vi "Agilent 428X Series Measure Capacitor D Value.vi"(7 "Voltage Level (V)(1.0V)":dbl=1.0 min=0.0 max=20.0 step=0.1 format="%.4f", 8 "error in (no error)":errorcluster, 9 "Freq Value (Hz)(1.0 MHz)":dbl=1000000.0 min=20.0 max=30000000.0 step=10.0 format="%.4e", 10 "Imp Type (0: CPD)":u32(ring) items=["CPD", "CPQ", "CPG", "CPRP", "CSD", "CSQ", "CSRS", "LPQ", "LPD", "LPG", "LPRP", "LSD", "LSQ", "LSRS", "RX", "ZTD", "ZTR", "GB", "YTD", "YTR"], 11 "VISA resource name":refnum<visa-resource-name>) -> (0 "error out":errorcluster, 1 "Secondary Value":dbl format="%^.4e", 2 "Primary Value":dbl format="%^.4e", 3 "VISA resource name out":refnum<visa-resource-name>, 4 "Data Status":bool=TRUE)   [LabVIEW 2015]
doc: "This VI is an example of how to use the HP428XA subVIs programmatically. This VI first configures a measurement, sets triggering, then takes measurements.\n\nThis function demonstrate one type of impedance measurement that can be made with the HP428XA and it accessories. In this example a 220 pF ceramic capacitor will be measured under the following conditions.\n\n DUT:\n 220 pF ceramic capacitor\n (HP Part Number 0160-4812)\n\n Measurement Conditions: \n \n Function: Cp-D\n Frequency: 1.0 MHz\n Test Signal Level: 1.0 V\n \n Equipment Required:\n\n HP 16047C Test Fixture\n Shorting bar (HP Part Number 5000-4226) or equivalent\n\nNote:\nFor more details see to the operation manual in Chapter 3."
uses:
  <instrlib>/Agilent 428X Series/Agilent 428X Series.lvlib
panel:
  # "© Copyright 2005 National Instruments Corporation.  All Rights Reserved."
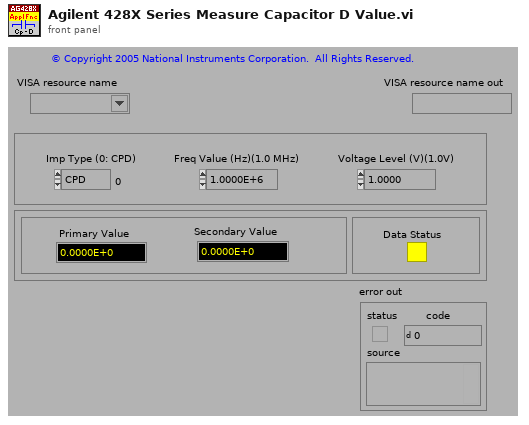
[diagram p1: front panel]
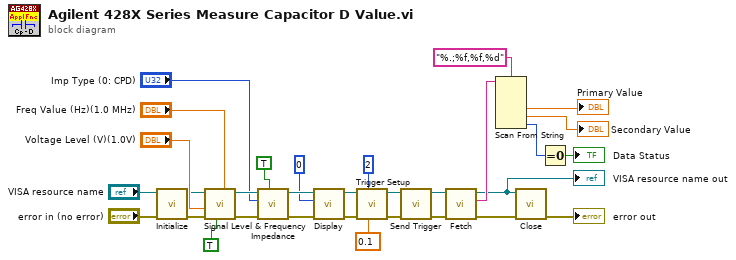
[diagram p0: block diagram]
diagram:
  n1 = call <instrlib>:"Initialize.vi"("error in (no error)"="error in (no error)", "VISA resource name"="VISA resource name") -> ("error out"=w5:errorcluster, "VISA resource name out"=w4:refnum<visa-resource-name>)  [unwired: 8 in]
  n2 = call <instrlib>:"Signal Level & Frequency.vi"("Frequency Value (Hz) (100KHz)"="Freq Value (Hz)(1.0 MHz)", "Oscillator Select (T: Voltage)"=TRUE, "error in (no error)"=w5, "Voltage Level (V) (5mV)"="Voltage Level (V)(1.0V)", "VISA resource name"=w4) -> ("error out"=w23:errorcluster, "VISA resource name out"=w31:refnum<visa-resource-name>)  [unwired: 5 in]
  n3 = call <instrlib>:"Impedance.vi"("Auto Range (F: Off)"=TRUE ("Auto Range (Off:F)"), "error in (no error)"=w23, "Imp Type (0: CPD)"="Imp Type (0: CPD)", "VISA resource name"=w31) -> ("error out"=w24:errorcluster, "VISA resource name out"=w30:refnum<visa-resource-name>)  [unwired: 6 in]
  n4 = call <instrlib>:"Display.vi"("error in (no error)"=w24, "Display Page (0: Measurement)"=u32 0 ("Display Page (Measurment:0)"), "VISA resource name"=w30) -> ("error out"=w25:errorcluster, "VISA resource name out"=w29:refnum<visa-resource-name>)  [unwired: 7 in]
  n5 = call <instrlib>:"Trigger Setup.vi"("Delay Value (s) (0.0)"=0.1, "Trigger Source (0: Internal)"=u32 2 ("Trigger Source (Internal:0)"), "error in (no error)"=w25, "VISA resource name"=w29) -> ("error out"=w26:errorcluster, "VISA resource name out"=w28:refnum<visa-resource-name>)  [unwired: 6 in]
  n6 = call <instrlib>:"Send Trigger.vi"("error in (no error)"=w26, "VISA resource name"=w28) -> ("error out"=w12:errorcluster, "VISA resource name out"=w27:refnum<visa-resource-name>)  [unwired: 8 in]
  n7 = call <instrlib>:"Fetch.vi"("error in (no error)"=w12, "VISA resource name"=w27) -> ("error out"=w3:errorcluster, "Returned Data"=w19:string, "VISA resource name out"=w1:refnum<visa-resource-name>)  [unwired: 7 in]
  "VISA resource name out" <- w1
  n8 = Scan From String(format string="%.;%f,%f,%d", input string=w19) -> (output 1=→"Primary Value":dbl, output 2=→"Secondary Value":dbl, output 3=w16:i32)  [unwired: 5 in, 3 out]
  n9 = call <instrlib>:"Close.vi"("error in (no error)"=w3, "VISA resource name"=w1) -> ("error out"=→"error out":errorcluster)  [unwired: 9 in]
  n10 = Equal To 0?(x=w16) -> (x = 0?=→"Data Status":bool)
